vi "He4 Mano Init.vi"   [LabVIEW 2019]
uses:
  TTM Global.vi
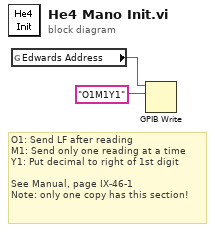
[diagram p0: block diagram]
diagram:
  # "O1: Send LF after reading\nM1: Send only one reading at a time\nY1: Put decimal to right of 1st digit\n\nSee Manual, page IX-46-1\nNote: only one copy has this section!"
  n1 = global read "TTM Global.vi" "Edwards Address"() -> (w1:string)
  n2 = GPIB Write(0:w1, 1:"O1M1Y1" ("data")) -> ()  [unwired: 3 in, 2 out]
